vi "Turbo Pump Controller 2.vi"() -> ()   [LabVIEW 2012]
panel:
  out "Voltage":u16=35604
  out "Current":dbl=35604.0
  out "Temperature":u16=35604
  out "Frequency":u16=35604
  out "Parameter":u32=35604
  out "Status Byte11&12":u16=35604 format="%04x"
  out "Pump Status":bool[](array[boolean])=[TRUE, FALSE, FALSE, FALSE, TRUE, FALSE, TRUE, TRUE, FALSE, FALSE, FALSE, TRUE, FALSE, TRUE, FALSE, FALSE]
  in  "Resend Command":bool
  out "Byte11&12":u16=1025 format="%04x"
  in  "USS Control Word (PZD1)":bool[](array[boolean])=[FALSE, FALSE, FALSE, FALSE, FALSE, TRUE, FALSE, FALSE, FALSE, FALSE, FALSE, FALSE, FALSE, FALSE, FALSE, TRUE]
  out "Telegram String":string
  in  "Param.  Value (Dez)":u32
  in  "Param.  Index (Dez)":u8
  out "Byte3&4":u16=4101 format="%04x"
  in  "Parameter Code (Dez)":u16=5
  out "Byte 3&4 (16 bits)":bool[](array[boolean])=[FALSE, FALSE, FALSE, TRUE, FALSE, FALSE, FALSE, FALSE, FALSE, FALSE, FALSE, FALSE, FALSE, TRUE, FALSE, TRUE]
  in  "Access Type":T1(ring)=enum."Parameter value requested"
  out "Telegram (24 bytes in Hex)":u8[](array[numeric])=[2, 22, 0, 16, 5, 0, 0, 0, 0, 0, 0, 4, 1, 0, 0, 0, 0, 0, 0, 0, 0, 0, 0, 4] format="%02x"
  in  "Send":bool
  out "Raw Reply":string
  # "For RS485 serial chanel communication with Leybold turbo pump"
  # "bit-15, 24 VDC output X203"
  # "bit-15, Process channel enabled"
  # "Byte 6 (IND)"
  # "bit-14, 24 VDC output X202"
  # "bit-14, Collective warning"
  # "Parameter Type and Adress (PKE)"
  # "bit-13, Warning relay X1"
  # "bit-13, Overload warning"
  # "bit-12, Normal operation relay X1"
  # "bit-12, No function"
  # "bit-15"
  # "bit-0"
  # "bit-11, Error operation relay X1"
  # "bit-11, Pump is turning"
  # "Byte 7-10 (PWE)"
  # "bit-10, Enable process data(bit 0,5-8,13-15)"
  # "bit-10, Normal operation detained"
  # "bit-9, Not assigned"
  # "bit-9, Parameter channel enabled"
  # "bit-8, Enable standby function"
  # "bit-8, No function"
  # "byte-0"
  # "byte-23"
  # "bit-7, Reset error (all components)"
  # "bit-7, Temperature warning"
  # "bit-6, Enable main setpoint PZD2"
  # "bit-6, Switch-on lock"
  # "bit-5, 24VDC output X201"
  # "bit-5, Decelerating"
  # "bit-4, Not assigned"
  # "bit-4, Accelerating"
  # "bit-3, Not assigned"
  # "bit-3, Error condition (all components)"
  # "bit-2, Not assigned"
  # "bit-2, Operation enabled"
  # "bit-1, Not assigned"
  # "bit-1, No function"
  # "bit-0, Start / Stop"
  # "bit-0, Ready for operation"
  # "(in Hex for byte 11&12)"
  # "(in Hex for byte 11&12)"
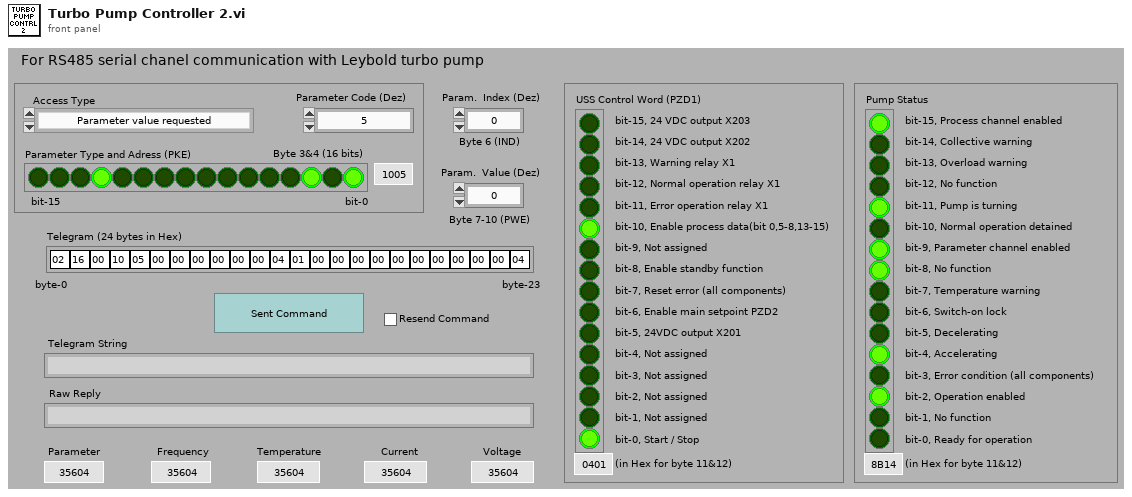
[diagram p1: front panel]
types:
  T1 = enum16{"No access", "Parameter value requested", "Write a16-bit value", "Write a 32-bit value", "Field value requested", "Write a 16-bit field value", "Write a 32-bit field value"}
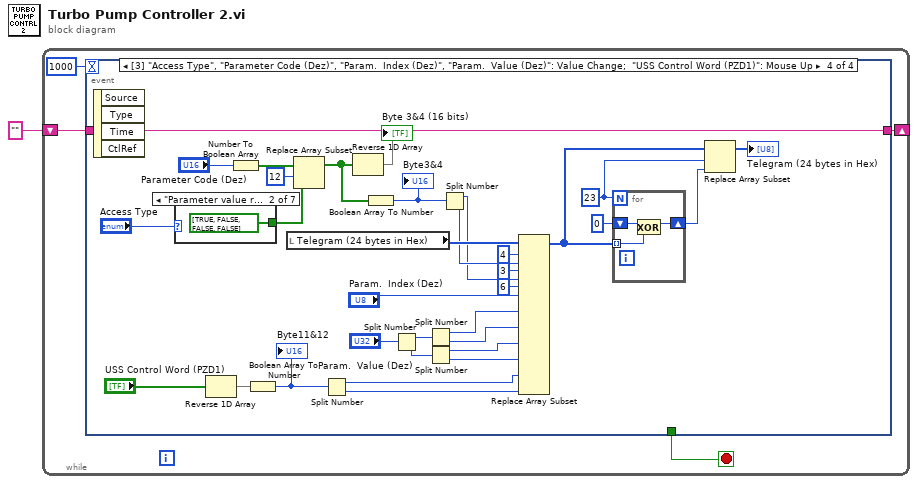
[diagram p0: block diagram]
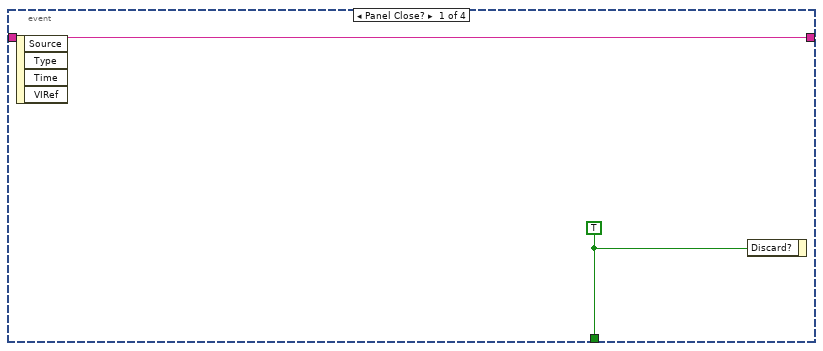
[diagram p2: hidden frame]
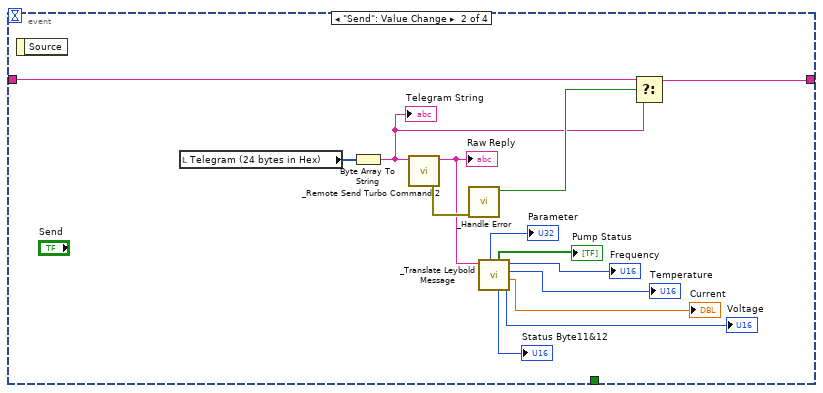
[diagram p3: hidden frame]
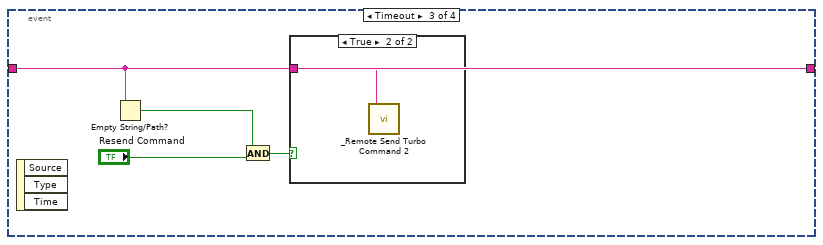
[diagram p4: hidden frame]
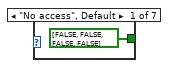
[diagram p6: hidden frame]
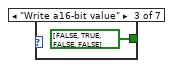
[diagram p7: hidden frame]
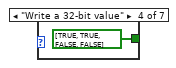
[diagram p8: hidden frame]
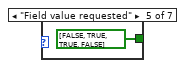
[diagram p9: hidden frame]
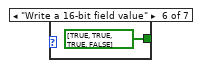
[diagram p10: hidden frame]
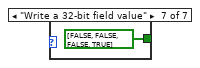
[diagram p11: hidden frame]
diagram:
  n1 = while {
    shift-right: [w3] -> _
    shift-left: "" -> [w4]
    stop <- w5 stop-if-true
    n2 = event shown="[3] \"Access Type\", \"Parameter Code (Dez)\", \"Param.  Index (Dez)\", \"Param.  Value (Dez)\": Value Change;  \"USS Control Word (PZD1)\": Mouse Up" {
      selector: _ -> [_ _ _ _]
      dyn-events: _ -> [_ _ _ _]
      timeout: 1000 -> [_ _ _ _]
      tunnel: [w7 _ _ _] -> w5
      tunnel: w4 -> [w6 w18 w22 w27]
      tunnel: [w6 w17 w22 w27] -> w3
      event Panel Close? {
        w7 = TRUE
        n3 = event-data() -> ()  [unwired: 5 out]
        n4 = event-data("Discard?"=w7) -> ()  [unwired: 1 in, 1 out]
      }
      event "Send": Value Change {
        n5 = event-data() -> ()  [unwired: 2 out]
        n6 = local read "Telegram (24 bytes in Hex)"() -> (w21:u8[])
        n7 = Byte Array To String(unsigned byte array=w21) -> (string=w16:string)
        "Telegram String" <- w16
        n8 = call "_Remote Send Turbo Command 2.vi"("Telegram"=w16) -> ("error out"=w20:errorcluster, "Raw Reply"=w15:string)  [unwired: 5 in]
        "Raw Reply" <- w15
        n9 = call "_Handle Error.vi"("error in (no error)"=w20) -> ("error?"=w19:bool)  [unwired: 2 in, 4 out]
        n10 = call "_Translate Leybold Message.vi"("LeyboldMessage"=w15) -> ("Voltage"=→"Voltage":u16, "Current"=→"Current":dbl, "Temperature"=→"Temperature":u16, "Frequency"=→"Frequency":u16, "Byte11&12"=→"Status Byte11&12":u16, "Pump Status"=→"Pump Status":bool[], "Parameter"=→"Parameter":u32)  [unwired: 3 in, 1 out]
        n11 = Select(t=w18, s=w19, f=w16) -> (s? t:f=w17:string)
      }
      event Timeout {
        n12 = event-data() -> ()  [unwired: 4 out]
        n13 = Empty String/Path?(string/path=w22) -> (empty?=w24:bool)
        n14 = And(x=w24, y="Resend Command") -> (x .and. y?=w23:bool)
        n15 = case shown="True" w23 {
          tunnel: w22 -> [_ w26]
          frame False {
          }
          frame True {
            n16 = call "_Remote Send Turbo Command 2.vi"("Telegram"=w26) -> ()  [unwired: 5 in, 2 out]
          }
        }
      }
      event "Access Type", "Parameter Code (Dez)", "Param.  Index (Dez)", "Param.  Value (Dez)": Value Change; "USS Control Word (PZD1)": Mouse Up {
        w35 = 23
        n17 = event-data() -> ()  [unwired: 5 out]
        n18 = case shown="\"Parameter value requested\"" "Access Type" {
          tunnel: [bool[] [FALSE, FALSE, FALSE, FALSE] ("Byte 3&4 (16 bits)") bool[] [TRUE, FALSE, FALSE, FALSE] ("Byte 3&4 (16 bits)") bool[] [FALSE, TRUE, FALSE, FALSE] ("Byte 3&4 (16 bits)") bool[] [TRUE, TRUE, FALSE, FALSE] ("Byte 3&4 (16 bits)") bool[] [FALSE, TRUE, TRUE, FALSE] ("Byte 3&4 (16 bits)") bool[] [TRUE, TRUE, TRUE, FALSE] ("Byte 3&4 (16 bits)") bool[] [FALSE, FALSE, FALSE, TRUE] ("Byte 3&4 (16 bits)")] -> w55
          frame "No access", Default {
          }
          frame "Parameter value requested" {
          }
          frame "Write a16-bit value" {
          }
          frame "Write a 32-bit value" {
          }
          frame "Field value requested" {
          }
          frame "Write a 16-bit field value" {
          }
          frame "Write a 32-bit field value" {
          }
        }
        n19 = Reverse 1D Array(array="USS Control Word (PZD1)") -> (reversed array=w28:bool[])
        n20 = Number To Boolean Array(number="Parameter Code (Dez)") -> (Boolean array=w57:bool[])
        n21 = Boolean Array To Number(Boolean array=w28) -> (number=w32:u16)
        "Byte11&12" <- w32
        n22 = local read "Telegram (24 bytes in Hex)"() -> (w53:u8[])
        n23 = Replace Array Subset(array=w57, new element=w55, index=12) -> (w47:bool[])
        n24 = Split Number(x=w32) -> (hi(x)=w31:u8, lo(x)=w30:u8)
        n25 = Reverse 1D Array(array=w47) -> (reversed array=→"Byte 3&4 (16 bits)":bool[])
        n26 = Boolean Array To Number(Boolean array=w47) -> (number=w54:u16)
        "Byte3&4" <- w54
        n27 = Split Number(x="Param.  Value (Dez)") -> (hi(x)=w42:u16, lo(x)=w43:u16)
        n28 = Split Number(x=w42) -> (hi(x)=w41:u8, lo(x)=w40:u8)
        n29 = Split Number(x=w43) -> (hi(x)=w39:u8, lo(x)=w38:u8)
        n30 = Split Number(x=w54) -> (hi(x)=w49:u8, lo(x)=w50:u8)
        n31 = Replace Array Subset(array=w53, new element #1=w50, index #1=4 ("index"), new element #2=w49, index #2=3 ("index"), new element #3="Param.  Index (Dez)", index #3=6 ("index"), new element #4=w41, new element #5=w40, new element #6=w39, new element #7=w38, new element #8=w31, new element #9=w30) -> (w36:u8[])  [unwired: 6 in]
        n32 = for {
          N: w35 -> [_]
          tunnel: w36 -> [w61] mode=indexing
          shift-right: [w60] -> w34
          shift-left: u8 0 -> [w62]
          n33 = Exclusive Or(1:w61, 2:w62) -> (0:w60:u8)
        }
        n34 = Replace Array Subset(array=w36, new element=w34, index=w35) -> (→"Telegram (24 bytes in Hex)":u8[])
      }
    }
  }
